vi "doubleshutter_imagesplit.vi"(3 "error in":errorcluster, 5 "image array":dbl[][](array[numeric]), 6 "Acquitsition Settings":T1) -> (0 "error out":errorcluster, 1 "upper half - background":dbl[][](graph), 2 "lower half - atoms":dbl[][](graph))   [LabVIEW 2016]
uses:
  Controls/PixelFly/Acquisition Settings.ctl
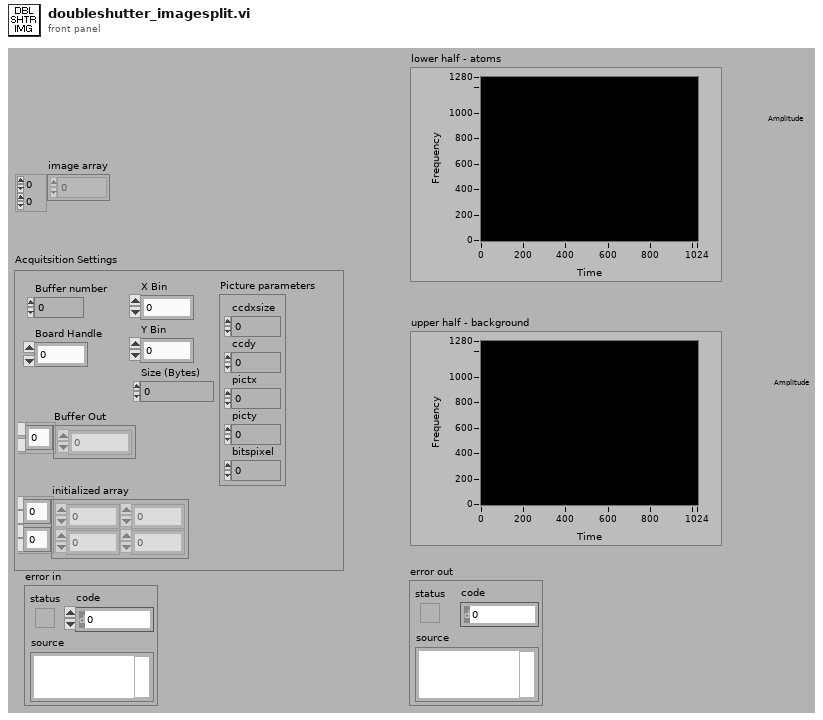
[diagram p1: front panel]
types:
  T1 = typedef "Acquisition Settings.ctl" = cluster{"Buffer number":i32, "Size (Bytes)":i32, "initialized array":u16[][], "X Bin":i32, "Y Bin":i32, "Board Handle":u32, "Picture parameters":cluster{"ccdxsize":i32, "ccdy":i32, "pictx":i32, "picty":i32, "bitspixel":i32}, "Buffer Out":u16[]}
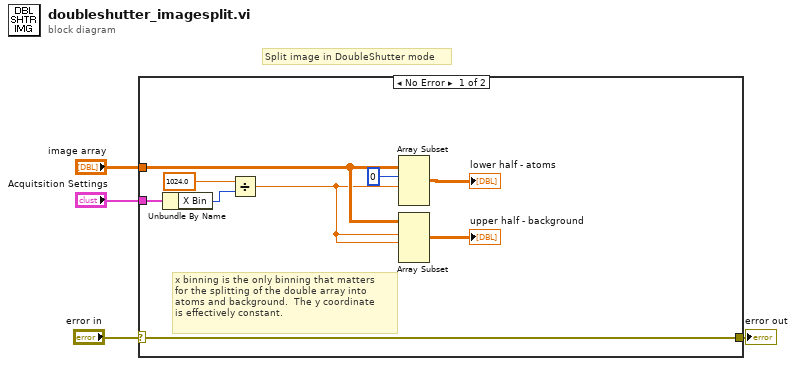
[diagram p0: block diagram]
diagram:
  # "Split image in DoubleShutter mode"
  n1 = case shown="No Error" "error in" {
    selector: "error in" -> [w7 w14]
    tunnel: "image array" -> [w13 _]
    tunnel: "Acquitsition Settings" -> [w9 _]
    tunnel: [w7 w14] -> w1
    frame No Error {
      # "x binning is the only binning that matters\nfor the splitting of the double array into\natoms and background.  The y coordinate\nis effectively constant."
      n2 = Unbundle By Name(w9) -> ("X Bin"=w8:i32)
      n3 = Divide(x=1024.0 ("length"), y=w8) -> (x/y=w10:dbl)
      n4 = Array Subset(array=w13, index (row)=0 ("index"), length (row)=w10) -> (→"lower half - atoms":dbl[][])  [unwired: 2 in]
      n5 = Array Subset(array=w13, index (row)=w10, length (row)=w10) -> (→"upper half - background":dbl[][])  [unwired: 2 in]
    }
    frame Error {
    }
  }
  "error out" <- w1
